vi "Configure Camera.vi"(8 "error in":errorcluster, 11 "IMG_SRC in":refnum<class "IMG_SRC.lvclass">) -> (0 "error out":errorcluster, 3 "IMG_SRC out":refnum<class "IMG_SRC.lvclass">)   [LabVIEW 2018, in "IMG_SRC.lvlib" / "IMG_SRC.lvclass"]
uses:
  IMG_SRC.lvclass
  IMG_SRC.lvclass/IMG_SRC.ctl
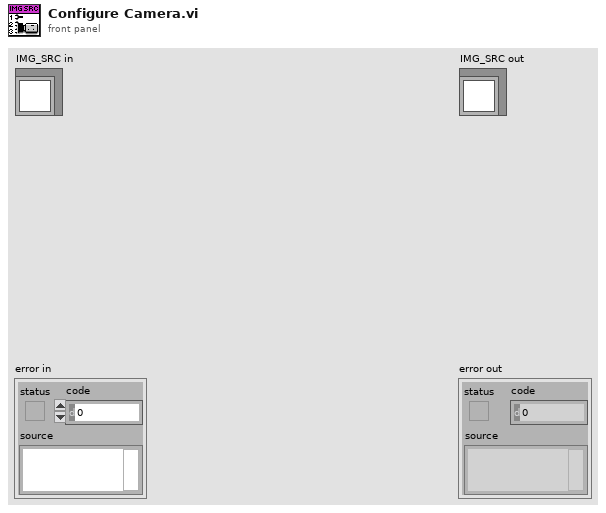
[diagram p1: front panel]
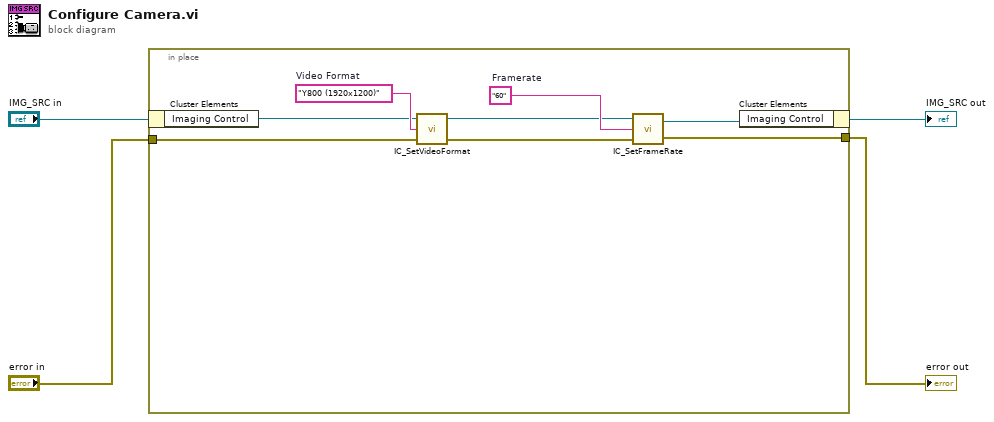
[diagram p0: block diagram]
diagram:
  n1 = in-place {
    in-place-border: [w6] -> w2
    in-place-border: "error in" -> [w5]
    w12 = "60"  # Framerate
    w11 = "Y800 (1920x1200)"  # Video Format
    n2 = in-place-cluster #1("IMG_SRC in") -> ("Imaging Control"=w10:refnum<k7>)
    n3 = call <userlib>:"IC_SetVideoFormat.vi"("Error In (no error)"=w5, "VideoFormat"=w11, "ICImagingControl In"=w10) -> ("Error Out"=w7:errorcluster, "ICImagingControl Out"=w9:refnum<k7>)  [unwired: 1 out]
    n4 = call <userlib>:"IC_SetFrameRate.vi"("Error In (no error)"=w7, "FrameRate"=w12, "ICImagingControl In"=w9) -> ("Error Out"=w6:errorcluster, "ICImagingControl Out"=w8:refnum<k7>)
    n5 = in-place-cluster #1("Imaging Control"=w8) -> (→"IMG_SRC out":refnum<class "IMG_SRC.lvclass">)
  }
  "error out" <- w2
